vi "climb with joysticks.vi"   [LabVIEW 2012]
uses:
  <vilib>/Rock Robotics/WPI/Solenoid/WPI_SolenoidValue.ctl
  Robot Global Data.vi
  <vilib>/Rock Robotics/WPI/Solenoid/WPI_SolenoidSetEnum.vi
types:
  T1 = typedef "WPI_JoystickButtonState.ctl" = cluster{"Button 1":bool, "Button 2":bool, "Button 3":bool, "Button 4":bool, "Button 5":bool, "Button 6":bool, "Button 7":bool, "Button 8":bool, "Button 9":bool, "Button 10":bool, "Button 11":bool, "Button 12":bool}
  T2 = typedef "WPI_ServoDeviceRef.ctl" = cluster{"DeviceStatus":errorcluster, "Digital Module":T3, "PWM Channel":T4, "DeadBand":T5}
  T3 = typedef "FPGA_TypedefDigitalModule.ctl" = enum16{"Digital Module 1", "Digital Module 2"}
  T4 = typedef "FPGA_DIOPWMChannel.ctl" = enum8{"PWM 1", "PWM 2", "PWM 3", "PWM 4", "PWM 5", "PWM 6", "PWM 7", "PWM 8", "PWM 9", "PWM 10", "Invalid"}
  T5 = typedef "WPI_PWMDeadband.ctl" = cluster{"Name":string, "maxPositivePwm":i32, "minPositivePwm":i32, "centerPwm":i32, "maxNegativePwm":i32, "minNegativePwm":i32, "angularRange":u16}
  T6 = typedef "WPI_SolenoidValue.ctl" = enum16{"Off", "On", "Forward", "Reverse"}
  T7 = typedef "WPI_SolenoidDevRef.ctl" = cluster{"DevStatus":errorcluster, "Solenoid Module":T8, "Forward Solenoid Channel":T9, "Reverse Solenoid Channel":T9}
  T8 = typedef "FPGA_TypedefSolenoidModule.ctl" = enum16{"Solenoid Module 1", "Solenoid Module 2"}
  T9 = typedef "WPI_SolenoidChannel.ctl" = enum8{"Solenoid 1", "Solenoid 2", "Solenoid 3", "Solenoid 4", "Solenoid 5", "Solenoid 6", "Solenoid 7", "Solenoid 8", "Invalid"}
  T10 = typedef "WPI_MotorControlDeviceRef.ctl" = cluster{"DeviceStatus":errorcluster, "Type":enum16{"PWM", "CAN"}, "PWM":cluster{"Digital Module":T3, "PWM Channel":T4, "DeadBand":T5}, "CAN":cluster{"Device Number":u8, "Control Mode":T11, "Semaphore":T12, "Max Vout":dbl}, "Invert":bool, "TransformRef":T13, "InvTransformRef":T13}
  T11 = typedef "WPI_CANJaguar_ControlMode.ctl" = enum8{"Percent VBus", "Current", "Speed", "Position", "Voltage"}
  T12 = typedef "Semaphore RefNum" = refnum<k1>
  T13 = typedef "WPI_PWMTransform_ConPane.ctl" = refnum<vi>
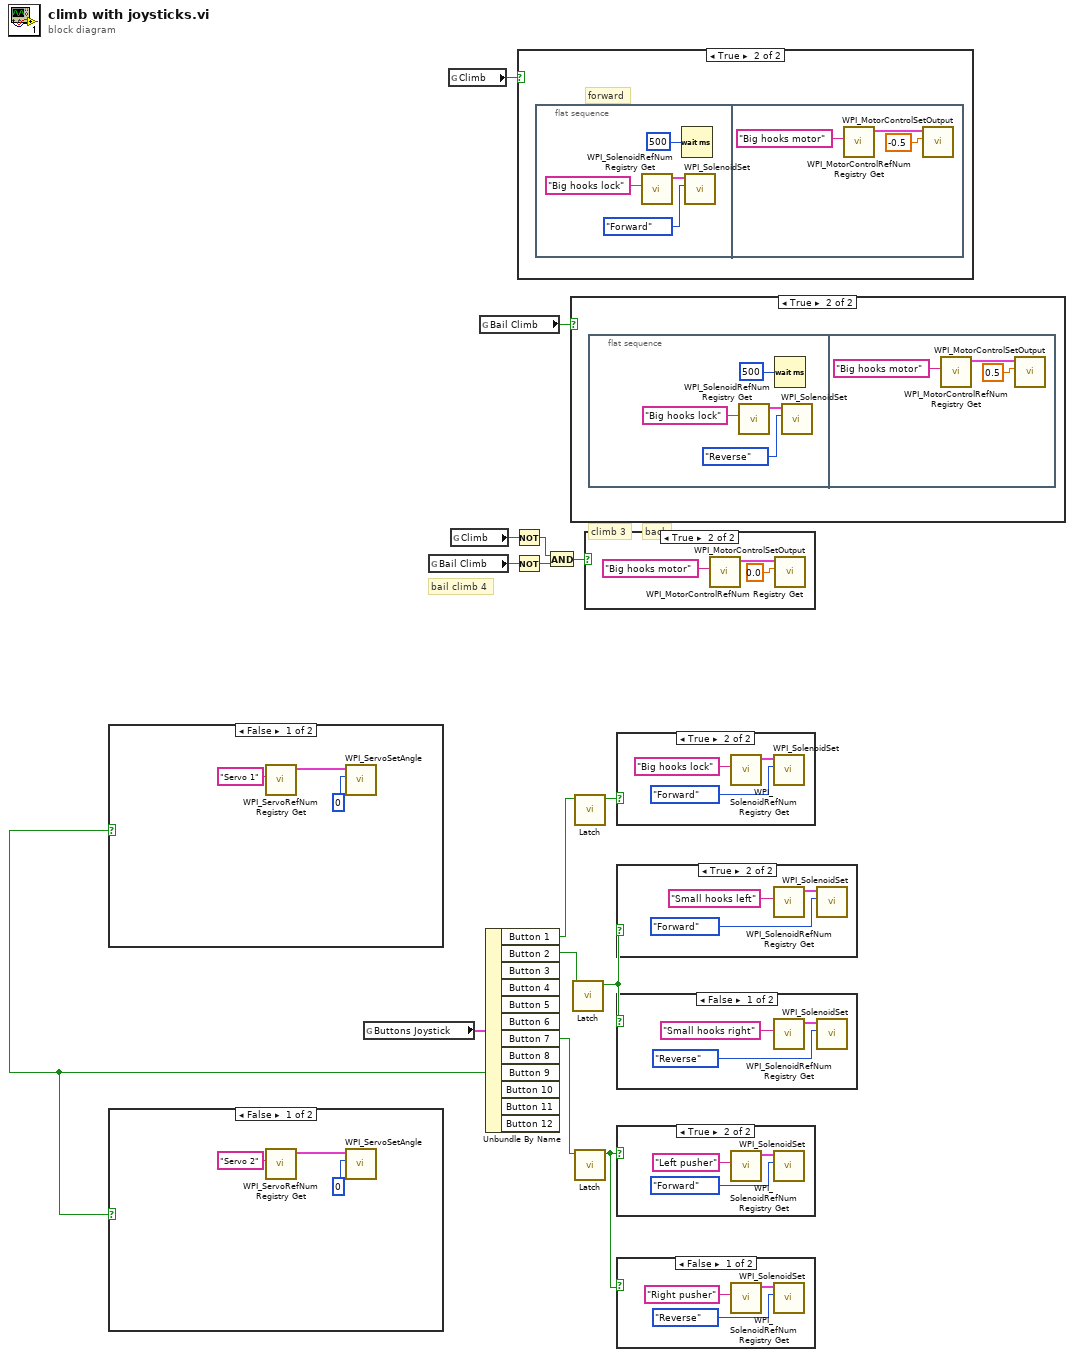
[diagram p0: block diagram]
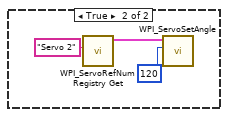
[diagram p2: hidden frame]
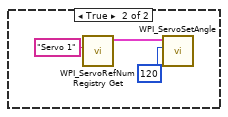
[diagram p3: hidden frame]
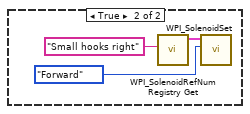
[diagram p4: hidden frame]
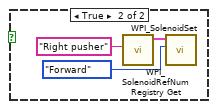
[diagram p5: hidden frame]
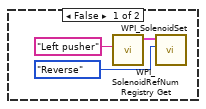
[diagram p6: hidden frame]
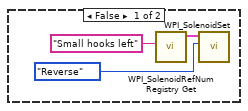
[diagram p7: hidden frame]
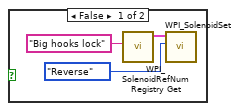
[diagram p8: hidden frame]
diagram:
  # "back"
  # "bail climb 4"
  # "climb 3"
  n1 = global read "Robot Global Data.vi" "Buttons Joystick"() -> (w8:T1)
  n2 = global read "Robot Global Data.vi" "Bail Climb"() -> (w10:bool)
  n3 = global read "Robot Global Data.vi" "Climb"() -> (w15:bool)
  n4 = global read "Robot Global Data.vi" "Climb"() -> (w12:bool)
  n5 = global read "Robot Global Data.vi" "Bail Climb"() -> (w14:bool)
  n6 = Unbundle By Name(w8) -> ("Button 1"=w7:bool, "Button 2"=w2:bool, "Button 7"=w5:bool, "Button 9"=w1:bool)  [unwired: 8 out]
  n7 = case shown="False" w1 {
    frame False {
      n8 = call <vilib>:"WPI_ServoRefNum Registry Get.vi"("refnum name"="Servo 1") -> ("ServoDeviceRef"=w18:T2)  [unwired: 9 in, 1 out]
      n9 = call <vilib>:"WPI_ServoSetAngle.vi"("Angle"=0, "ServoDeviceRef"=w18) -> ()  [unwired: 8 in, 2 out]
    }
    frame True {
      n10 = call <vilib>:"WPI_ServoRefNum Registry Get.vi"("refnum name"="Servo 1") -> ("ServoDeviceRef"=w21:T2)  [unwired: 9 in, 1 out]
      n11 = call <vilib>:"WPI_ServoSetAngle.vi"("Angle"=120, "ServoDeviceRef"=w21) -> ()  [unwired: 8 in, 2 out]
    }
  }
  n12 = case shown="False" w1 {
    frame False {
      n13 = call <vilib>:"WPI_ServoRefNum Registry Get.vi"("refnum name"="Servo 2") -> ("ServoDeviceRef"=w24:T2)  [unwired: 9 in, 1 out]
      n14 = call <vilib>:"WPI_ServoSetAngle.vi"("Angle"=0, "ServoDeviceRef"=w24) -> ()  [unwired: 8 in, 2 out]
    }
    frame True {
      n15 = call <vilib>:"WPI_ServoRefNum Registry Get.vi"("refnum name"="Servo 2") -> ("ServoDeviceRef"=w27:T2)  [unwired: 9 in, 1 out]
      n16 = call <vilib>:"WPI_ServoSetAngle.vi"("Angle"=120, "ServoDeviceRef"=w27) -> ()  [unwired: 8 in, 2 out]
    }
  }
  n17 = Not(x=w12) -> (.not. x?=w11:bool)
  n18 = Not(x=w10) -> (.not. x?=w9:bool)
  n19 = case shown="True" w15 {
    frame False {
    }
    frame True {
      # "forward"
      n20 = flat-sequence {
        frame #0 {
          n21 = call <vilib>:"WPI_SolenoidRefNum Registry Get.vi"("refnum name"="Big hooks lock") -> ("SolenoidDevRef"=w30:T7)  [unwired: 9 in, 1 out]
          n22 = Wait (ms)(milliseconds to wait=u32 500) -> ()  [unwired: 1 out]
          n23 = call-poly <vilib>:"WPI_SolenoidSet.vi"("Value"=WPI_SolenoidValue."Forward", "SolenoidDevRef"=w30) -> ()  [unwired: 8 in, 2 out]
        }
        frame #1 {
          n24 = call <vilib>:"WPI_MotorControlRefNum Registry Get.vi"("refnum name"="Big hooks motor") -> ("MotorControlDevRef"=w34:T10)  [unwired: 9 in, 1 out]
          n25 = call <vilib>:"WPI_MotorControlSetOutput.vi"("Output"=-0.5, "MotorControlDevRef"=w34) -> ()  [unwired: 7 in, 3 out]
        }
      }
    }
  }
  n26 = And(x=w11, y=w9) -> (x .and. y?=w13:bool)
  n27 = case shown="True" w14 {
    frame False {
    }
    frame True {
      n28 = flat-sequence {
        frame #0 {
          n29 = call <vilib>:"WPI_SolenoidRefNum Registry Get.vi"("refnum name"="Big hooks lock") -> ("SolenoidDevRef"=w37:T7)  [unwired: 9 in, 1 out]
          n30 = Wait (ms)(milliseconds to wait=u32 500) -> ()  [unwired: 1 out]
          n31 = call-poly <vilib>:"WPI_SolenoidSet.vi"("Value"=WPI_SolenoidValue."Reverse", "SolenoidDevRef"=w37) -> ()  [unwired: 8 in, 2 out]
        }
        frame #1 {
          n32 = call <vilib>:"WPI_MotorControlRefNum Registry Get.vi"("refnum name"="Big hooks motor") -> ("MotorControlDevRef"=w41:T10)  [unwired: 9 in, 1 out]
          n33 = call <vilib>:"WPI_MotorControlSetOutput.vi"("Output"=0.5, "MotorControlDevRef"=w41) -> ()  [unwired: 7 in, 3 out]
        }
      }
    }
  }
  n34 = call "Latch.vi"("Input"=w2) -> ("Output"=w4:bool)  [unwired: 9 in]
  n35 = call "Latch.vi"("Input"=w7) -> ("Output"=w6:bool)  [unwired: 9 in]
  n36 = call "Latch.vi"("Input"=w5) -> ("Output"=w3:bool)  [unwired: 9 in]
  n37 = case shown="True" w13 {
    frame False {
    }
    frame True {
      n38 = call <vilib>:"WPI_MotorControlRefNum Registry Get.vi"("refnum name"="Big hooks motor") -> ("MotorControlDevRef"=w44:T10)  [unwired: 9 in, 1 out]
      n39 = call <vilib>:"WPI_MotorControlSetOutput.vi"("Output"=0.0, "MotorControlDevRef"=w44) -> ()  [unwired: 7 in, 3 out]
    }
  }
  n40 = case shown="True" w6 {
    frame False {
      n41 = call <vilib>:"WPI_SolenoidRefNum Registry Get.vi"("refnum name"="Big hooks lock") -> ("SolenoidDevRef"=w46:T7)  [unwired: 9 in, 1 out]
      n42 = call-poly <vilib>:"WPI_SolenoidSet.vi"("Value"=WPI_SolenoidValue."Reverse", "SolenoidDevRef"=w46) -> ()  [unwired: 8 in, 2 out]
    }
    frame True {
      n43 = call <vilib>:"WPI_SolenoidRefNum Registry Get.vi"("refnum name"="Big hooks lock") -> ("SolenoidDevRef"=w49:T7)  [unwired: 9 in, 1 out]
      n44 = call-poly <vilib>:"WPI_SolenoidSet.vi"("Value"=WPI_SolenoidValue."Forward", "SolenoidDevRef"=w49) -> ()  [unwired: 8 in, 2 out]
    }
  }
  n45 = case shown="True" w4 {
    frame False {
      n46 = call <vilib>:"WPI_SolenoidRefNum Registry Get.vi"("refnum name"="Small hooks left") -> ("SolenoidDevRef"=w52:T7)  [unwired: 9 in, 1 out]
      n47 = call-poly <vilib>:"WPI_SolenoidSet.vi"("Value"=WPI_SolenoidValue."Reverse", "SolenoidDevRef"=w52) -> ()  [unwired: 8 in, 2 out]
    }
    frame True {
      n48 = call <vilib>:"WPI_SolenoidRefNum Registry Get.vi"("refnum name"="Small hooks left") -> ("SolenoidDevRef"=w55:T7)  [unwired: 9 in, 1 out]
      n49 = call-poly <vilib>:"WPI_SolenoidSet.vi"("Value"=WPI_SolenoidValue."Forward", "SolenoidDevRef"=w55) -> ()  [unwired: 8 in, 2 out]
    }
  }
  n50 = case shown="False" w4 {
    frame False {
      n51 = call <vilib>:"WPI_SolenoidRefNum Registry Get.vi"("refnum name"="Small hooks right") -> ("SolenoidDevRef"=w58:T7)  [unwired: 9 in, 1 out]
      n52 = call-poly <vilib>:"WPI_SolenoidSet.vi"("Value"=WPI_SolenoidValue."Reverse", "SolenoidDevRef"=w58) -> ()  [unwired: 8 in, 2 out]
    }
    frame True {
      n53 = call <vilib>:"WPI_SolenoidRefNum Registry Get.vi"("refnum name"="Small hooks right") -> ("SolenoidDevRef"=w61:T7)  [unwired: 9 in, 1 out]
      n54 = call-poly <vilib>:"WPI_SolenoidSet.vi"("Value"=WPI_SolenoidValue."Forward", "SolenoidDevRef"=w61) -> ()  [unwired: 8 in, 2 out]
    }
  }
  n55 = case shown="True" w3 {
    frame False {
      n56 = call <vilib>:"WPI_SolenoidRefNum Registry Get.vi"("refnum name"="Left pusher") -> ("SolenoidDevRef"=w64:T7)  [unwired: 9 in, 1 out]
      n57 = call-poly <vilib>:"WPI_SolenoidSet.vi"("Value"=WPI_SolenoidValue."Reverse", "SolenoidDevRef"=w64) -> ()  [unwired: 8 in, 2 out]
    }
    frame True {
      n58 = call <vilib>:"WPI_SolenoidRefNum Registry Get.vi"("refnum name"="Left pusher") -> ("SolenoidDevRef"=w67:T7)  [unwired: 9 in, 1 out]
      n59 = call-poly <vilib>:"WPI_SolenoidSet.vi"("Value"=WPI_SolenoidValue."Forward", "SolenoidDevRef"=w67) -> ()  [unwired: 8 in, 2 out]
    }
  }
  n60 = case shown="False" w3 {
    frame False {
      n61 = call <vilib>:"WPI_SolenoidRefNum Registry Get.vi"("refnum name"="Right pusher") -> ("SolenoidDevRef"=w70:T7)  [unwired: 9 in, 1 out]
      n62 = call-poly <vilib>:"WPI_SolenoidSet.vi"("Value"=WPI_SolenoidValue."Reverse", "SolenoidDevRef"=w70) -> ()  [unwired: 8 in, 2 out]
    }
    frame True {
      n63 = call <vilib>:"WPI_SolenoidRefNum Registry Get.vi"("refnum name"="Right pusher") -> ("SolenoidDevRef"=w73:T7)  [unwired: 9 in, 1 out]
      n64 = call-poly <vilib>:"WPI_SolenoidSet.vi"("Value"=WPI_SolenoidValue."Forward", "SolenoidDevRef"=w73) -> ()  [unwired: 8 in, 2 out]
    }
  }
